vi "ControlArmReadFromWebsite.vi"() -> ()   [LabVIEW 2024]
uses:
  <vilib>/httpClient/LabVIEWHTTPClient.lvlib
panel:
  out "body":string
  in  "stop":bool
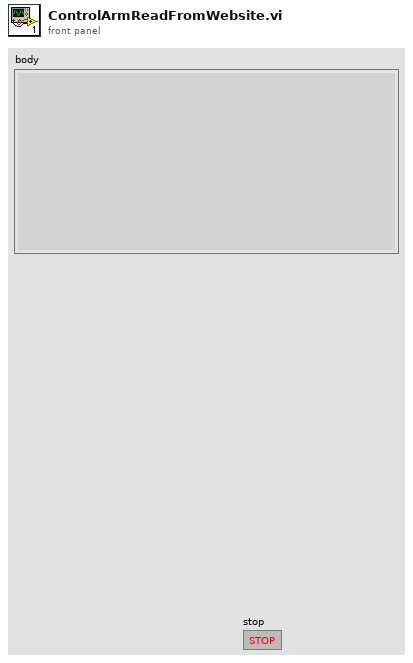
[diagram p1: front panel]
types:
  T1 = typedef "LabVIEWHTTPClient.lvlib/ClientHandle.ctl" = refnum<k1>
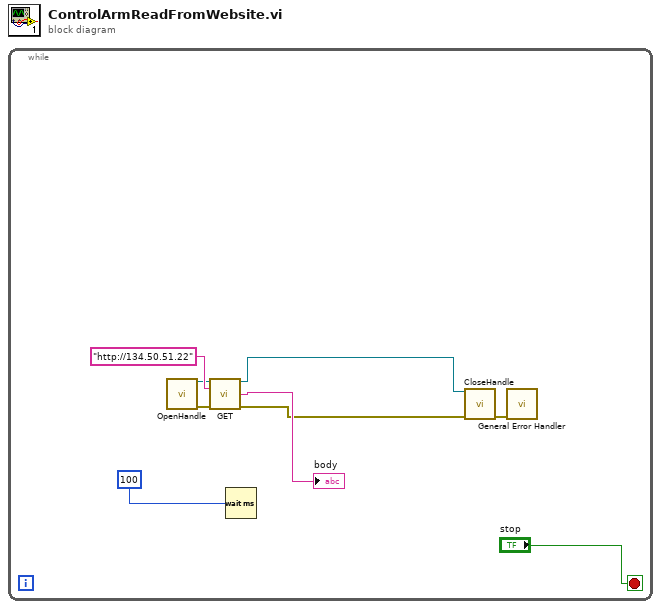
[diagram p0: block diagram]
diagram:
  n1 = while {
    stop <- "stop" stop-if-true
    n2 = call <vilib>:"OpenHandle.vi"() -> ("client handle out"=w8:T1, "error out"=w7:errorcluster)  [unwired: 14 in]
    n3 = call <vilib>:"GET.vi"("client handle"=w8, "url"="http://134.50.51.22", "error in (no error)"=w7) -> ("client handle out"=w5:T1, "body"=→"body":string, "error out"=w1:errorcluster)  [unwired: 9 in, 1 out]
    n4 = Wait (ms)(milliseconds to wait=u32 100) -> ()  [unwired: 1 out]
    n5 = call <vilib>:"CloseHandle.vi"("client handle"=w5, "error in (no error)"=w1) -> ("error out"=w6:errorcluster)  [unwired: 13 in]
    n6 = call <vilib>:"General Error Handler.vi"("error in (no error)"=w6) -> ()  [unwired: 10 in, 5 out]
  }
